vi "Test_ReadInconsistantSpreadsheet.vi"() -> ()   [LabVIEW 2014]
uses:
  functions/Timer_Global_Action_Control.ctl
panel:
  out "Time Difference 2":dbl
  out "Array Numeric":u8[](array[numeric])
  out "text":string
  out "Time Difference":dbl
  in  "type (empty)":string[][](array[string])
  out "all rows":string[][](array[string])
  # "10Mio Loops\n4,7sec"
  # "1k Loops:\nRaw: 0.0009999sec\nSmart: 14,1148sec"
  # "aa b   c\n\n#param1\tparam2\tparam3\tparam4\n!param5    param6\tparam7\tparam8\n\n1.00  1.20     1.30         1.40\n 2.00\t2.20\t2.30\t2.40\n3.00\t3.20\t3.30\t3.40\n     4.00    4.20   4.30 4.40"
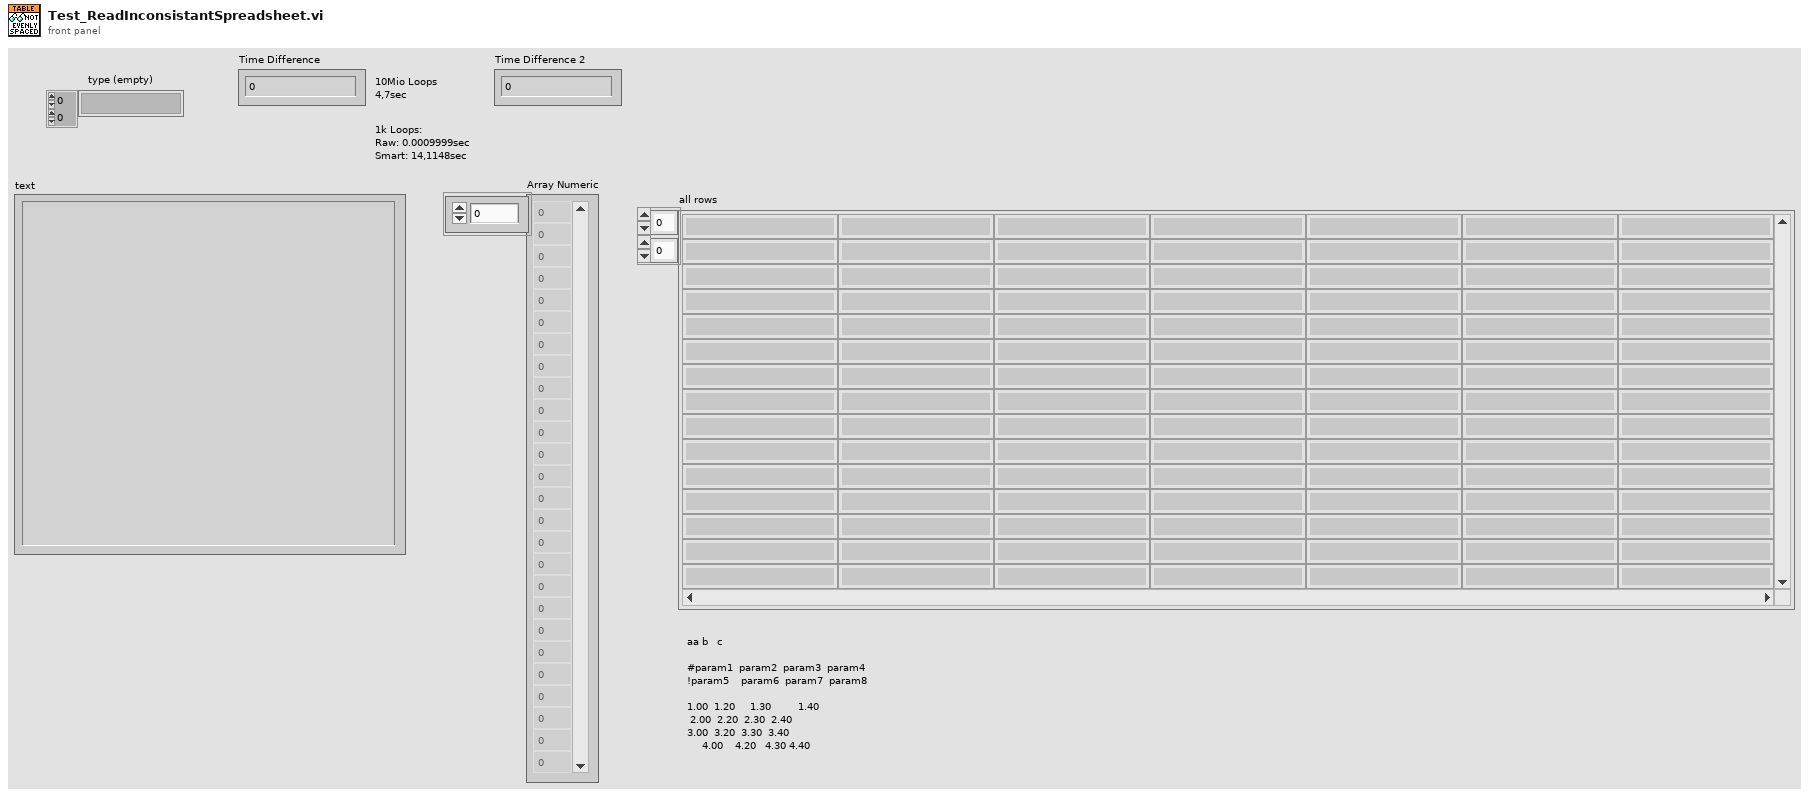
[diagram p1: front panel]
types:
  T1 = typedef "Timer_Global_Action_Control.ctl" = enum16{"Init", "Set", "Get", "Update", "Clear"}
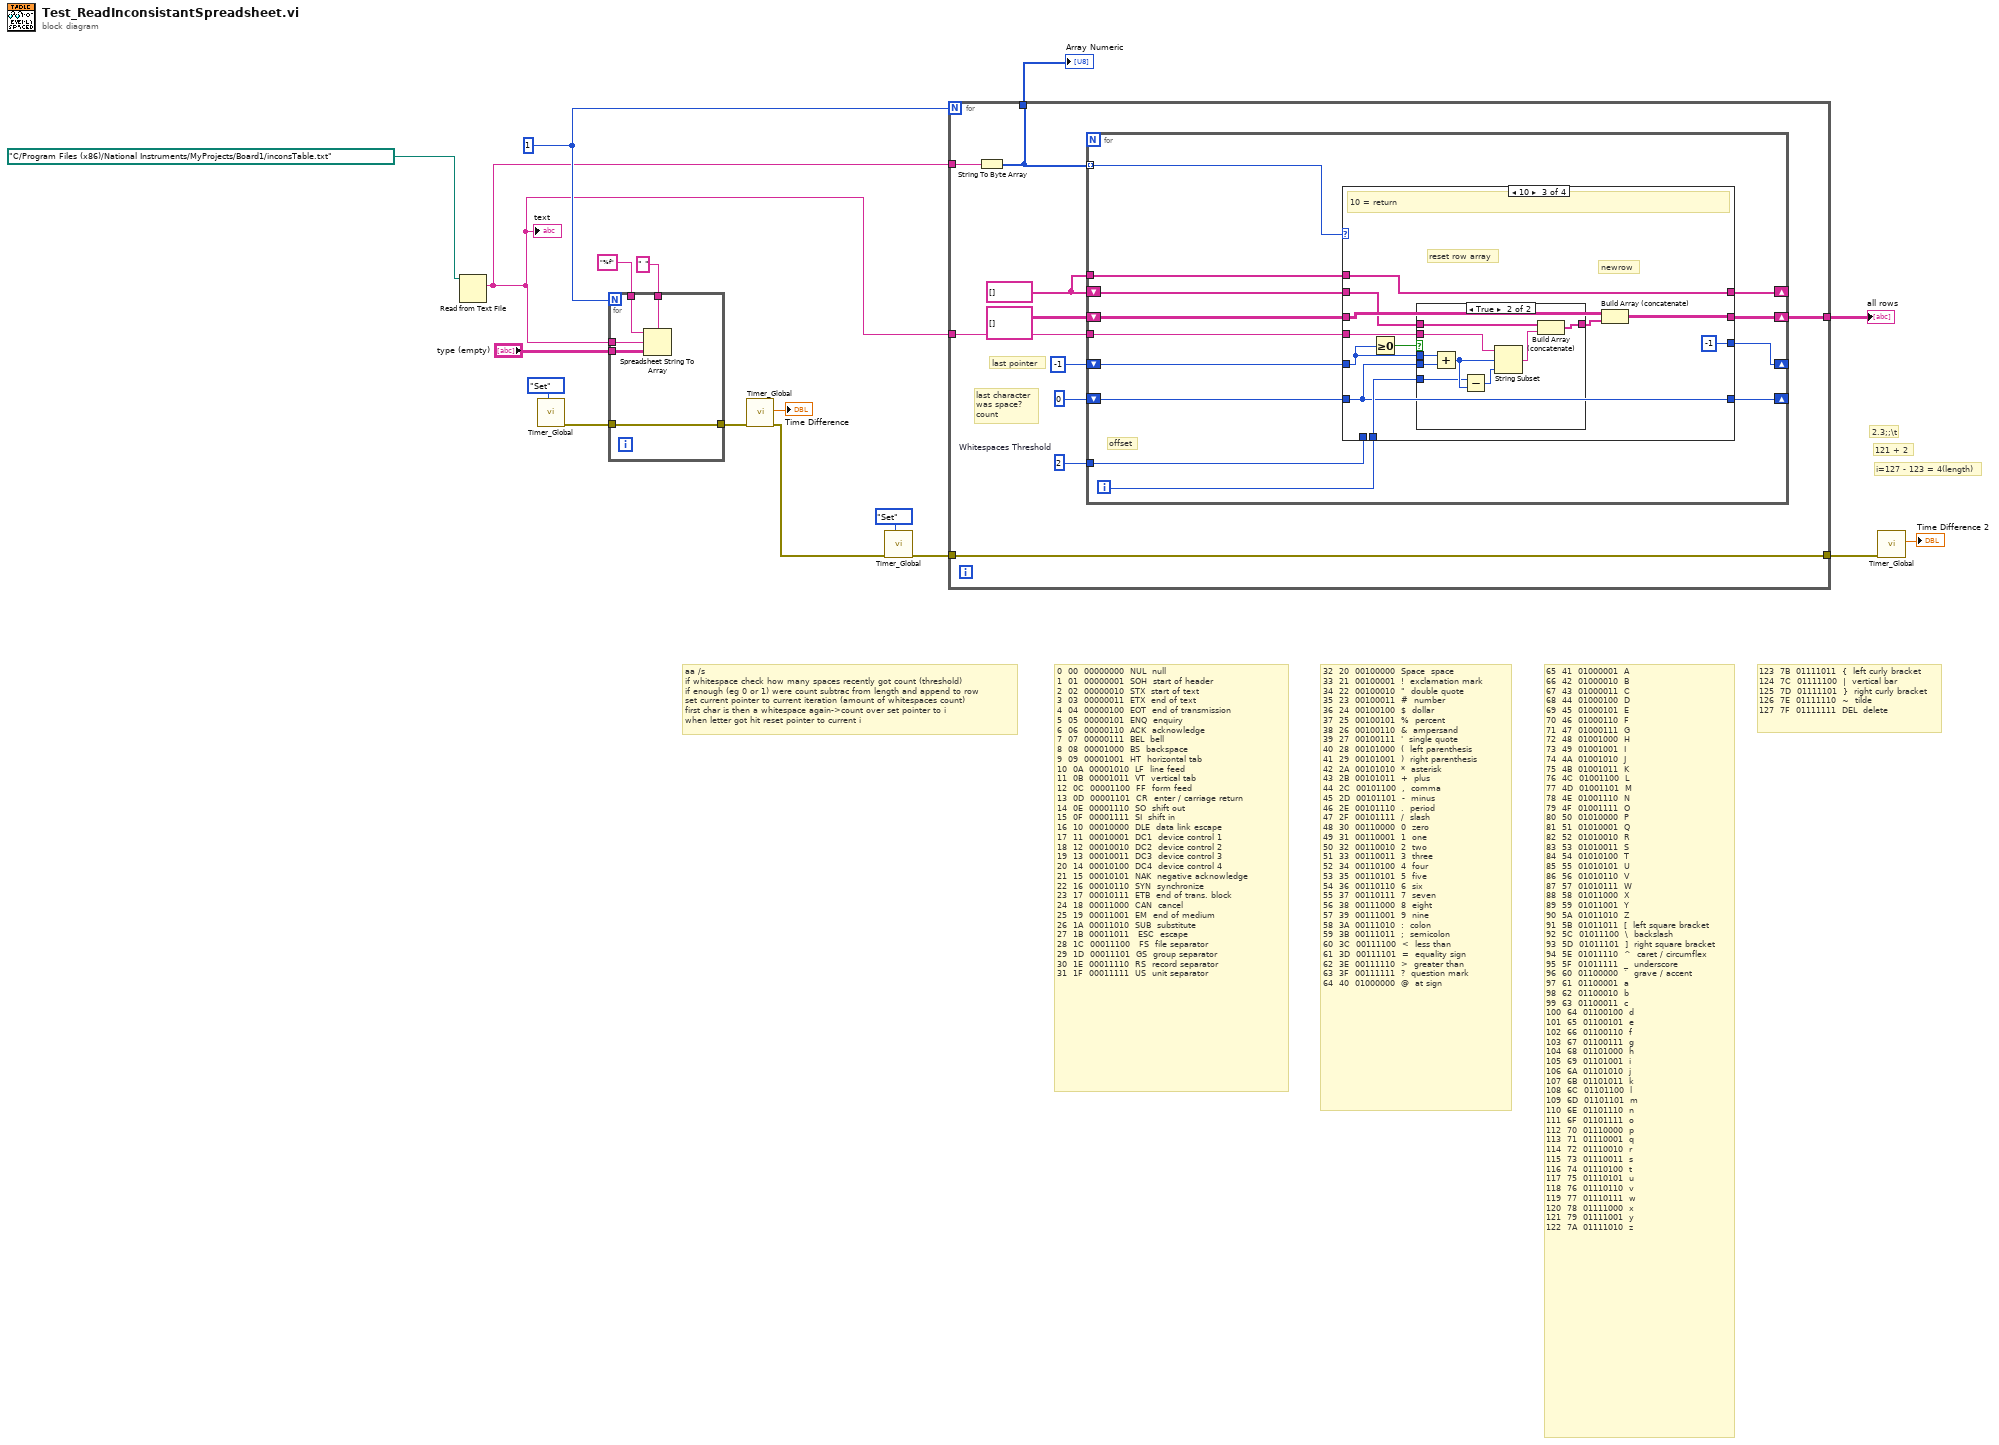
[diagram p0: block diagram]
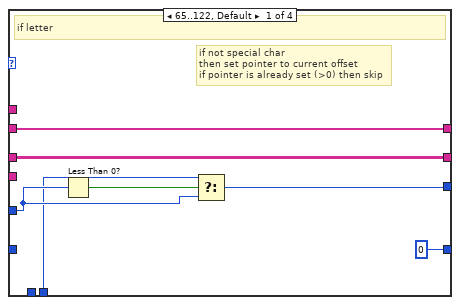
[diagram p2: hidden frame]
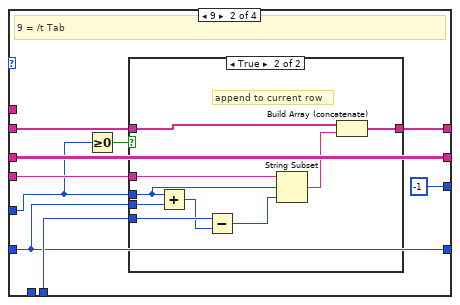
[diagram p3: hidden frame]
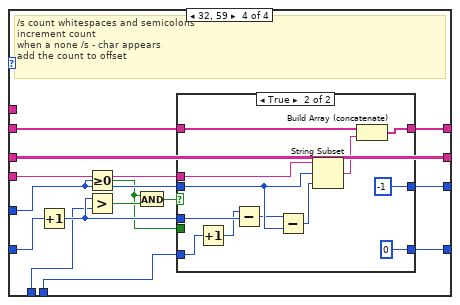
[diagram p6: hidden frame]
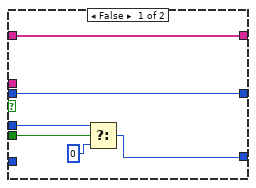
[diagram p7: hidden frame]
diagram:
  w3 = 1
  # "i=127 - 123 = 4(length)"
  # "121 + 2"
  # "2.3;;\\t"
  # "aa /s\nif whitespace check how many spaces recently got count (threshold)\nif enough (eg 0 or 1) were count subtrac from length and append to row\nset current pointer to current iteration (amount of whitespaces count)\nfirst char is then a whitespace again->count over set pointer to i\nwhen letter got hit reset pointer to current i"
  # "123 \t7B \t01111011 \t{ \tleft curly bracket\n124 \t7C \t01111100 \t| \tvertical bar\n125 \t7D \t01111101 \t} \tright curly bracket\n126 \t7E \t01111110 \t~ \ttilde\n127 \t7F \t01111111 \tDEL \tdelete"
  # "65 \t41 \t01000001 \tA \t \n66 \t42 \t01000010 \tB \t \n67 \t43 \t01000011 \tC \t \n68 \t44 \t01000100 \tD \t \n69 \t45 \t01000101 \tE \t \n70 \t46 \t01000110 \tF \t \n71 \t47 \t01000111 \tG \t \n72 \t48 \t01001000 \tH \t \n73 \t49 \t01001001 \tI \t \n74 \t4A \t01001010 \tJ \t \n75 \t4B \t01001011 \tK \t \n76 \t4C \t01001100 \tL \t \n77 \t4D \t01001101 \tM \t \n78 \t4E \t01001110 \tN \t \n79 \t4F \t01001111 \tO \t \n80 \t50 \t01010000 \tP \t \n81 \t51 \t01010001 \tQ \t \n82 \t52 \t01010010 \tR \t \n83 \t53 \t01010011 \tS \t \n84 \t54 \t01010100 \tT \t \n85 \t55 \t01010101 \tU \t \n86 \t56 \t01010110 \tV \t \n87 \t57 \t01010111 \tW \t \n88 \t58 \t01011000 \tX \t \n89 \t59 \t01011001 \tY \t \n90 \t5A \t01011010 \tZ \t \n91 \t5B \t01011011 \t[ \tleft square bracket\n92 \t5C \t01011100 \t\\ \tbackslash\n93 \t5D \t01011101 \t] \tright square bracket\n94 \t5E \t01011110 \t^ \tcaret / circumflex\n95 \t5F \t01011111 \t_ \tunderscore\n96 \t60 \t01100000 \t` \tgrave / accent\n97 \t61 \t01100001 \ta \t \n98 \t62 \t01100010 \tb \t \n99 \t63 \t01100011 \tc \t \n100 \t64 \t01100100 \td \t \n101 \t65 \t01100101 \te \t \n102 \t66 \t01100110 \tf \t \n103 \t67 \t01100111 \tg \t \n104 \t68 \t01101000 \th \t \n105 \t69 \t01101001 \ti \t \n106 \t6A \t01101010 \tj \t \n107 \t6B \t01101011 \tk \t \n108 \t6C \t01101100 \tl \t \n109 \t6D \t01101101 \tm \t \n110 \t6E \t01101110 \tn \t \n111 \t6F \t01101111 \to \t \n112 \t70 \t01110000 \tp \t \n113 \t71 \t01110001 \tq \t \n114 \t72 \t01110010 \tr \t \n115 \t73 \t01110011 \ts \t \n116 \t74 \t01110100 \tt \t \n117 \t75 \t01110101 \tu \t \n118 \t76 \t01110110 \tv \t \n119 \t77 \t01110111 \tw \t \n120 \t78 \t01111000 \tx \t \n121 \t79 \t01111001 \ty \t \n122 \t7A \t01111010 \tz"
  # "32 \t20 \t00100000 \tSpace \tspace\n33 \t21 \t00100001 \t! \texclamation mark\n34 \t22 \t00100010 \t\" \tdouble quote\n35 \t23 \t00100011 \t# \tnumber\n36 \t24 \t00100100 \t$ \tdollar\n37 \t25 \t00100101 \t% \tpercent\n38 \t26 \t00100110 \t& \tampersand\n39 \t27 \t00100111 \t' \tsingle quote\n40 \t28 \t00101000 \t( \tleft parenthesis\n41 \t29 \t00101001 \t) \tright parenthesis\n42 \t2A \t00101010 \t* \tasterisk\n43 \t2B \t00101011 \t+ \tplus\n44 \t2C \t00101100 \t, \tcomma\n45 \t2D \t00101101 \t- \tminus\n46 \t2E \t00101110 \t. \tperiod\n47 \t2F \t00101111 \t/ \tslash\n48 \t30 \t00110000 \t0 \tzero\n49 \t31 \t00110001 \t1 \tone\n50 \t32 \t00110010 \t2 \ttwo\n51 \t33 \t00110011 \t3 \tthree\n52 \t34 \t00110100 \t4 \tfour\n53 \t35 \t00110101 \t5 \tfive\n54 \t36 \t00110110 \t6 \tsix\n55 \t37 \t00110111 \t7 \tseven\n56 \t38 \t00111000 \t8 \teight\n57 \t39 \t00111001 \t9 \tnine\n58 \t3A \t00111010 \t: \tcolon\n59 \t3B \t00111011 \t; \tsemicolon\n60 \t3C \t00111100 \t< \tless than\n61 \t3D \t00111101 \t= \tequality sign\n62 \t3E \t00111110 \t> \tgreater than\n63 \t3F \t00111111 \t? \tquestion mark\n64 \t40 \t01000000 \t@ \tat sign"
  # "0 \t00 \t00000000 \tNUL \tnull\n1 \t01 \t00000001 \tSOH \tstart of header\n2 \t02 \t00000010 \tSTX \tstart of text\n3 \t03 \t00000011 \tETX \tend of text\n4 \t04 \t00000100 \tEOT \tend of transmission\n5 \t05 \t00000101 \tENQ \tenquiry\n6 \t06 \t00000110 \tACK \tacknowledge\n7 \t07 \t00000111 \tBEL \tbell\n8 \t08 \t00001000 \tBS \tbackspace\n9 \t09 \t00001001 \tHT \thorizontal tab\n10 \t0A \t00001010 \tLF \tline feed\n11 \t0B \t00001011 \tVT \tvertical tab\n12 \t0C \t00001100 \tFF \tform feed\n13 \t0D \t00001101 \tCR \tenter / carriage return\n14 \t0E \t00001110 \tSO \tshift out\n15 \t0F \t00001111 \tSI \tshift in\n16 \t10 \t00010000 \tDLE \tdata link escape\n17 \t11 \t00010001 \tDC1 \tdevice control 1\n18 \t12 \t00010010 \tDC2 \tdevice control 2\n19 \t13 \t00010011 \tDC3 \tdevice control 3\n20 \t14 \t00010100 \tDC4 \tdevice control 4\n21 \t15 \t00010101 \tNAK \tnegative acknowledge\n22 \t16 \t00010110 \tSYN \tsynchronize\n23 \t17 \t00010111 \tETB \tend of trans. block\n24 \t18 \t00011000 \tCAN \tcancel\n25 \t19 \t00011001 \tEM \tend of medium\n26 \t1A \t00011010 \tSUB \tsubstitute\n27 \t1B \t00011011 \t ESC \tescape\n28 \t1C \t00011100 \t FS \tfile separator\n29 \t1D \t00011101 \tGS \tgroup separator\n30 \t1E \t00011110 \tRS \trecord separator\n31 \t1F \t00011111 \tUS \tunit separator"
  n1 = Read from Text File(file (use dialog)=path "C:/Program Files (x86)/National Instruments/MyProjects/Board1/inconsTable.txt" ("Open File")) -> (text=w2:string)  [unwired: 3 in, 3 out]
  "text" <- w2
  n2 = call "Timer_Global.vi"("Timer Action"=Timer_Global_Action_Control."Set") -> ("Error Out"=w15:errorcluster)  [unwired: 8 in, 2 out]
  n3 = for {
    N: w3 -> [_]
    tunnel: "type (empty)" -> [w22]
    tunnel: w2 -> [w19]
    tunnel: [w21] -> w14
    tunnel: w15 -> [w21]
    tunnel: " " ("delimiter (\\t)") -> [w20]
    tunnel: "%f" ("format (%s)") -> [w18]
    n4 = Spreadsheet String To Array(delimiter (Tab)=w20, format string=w18, spreadsheet string=w19, array type (2D Dbl)=w22) -> ()  [unwired: 1 out]
  }
  n5 = call "Timer_Global.vi"("Error In"=w14) -> ("Error Out"=w7:errorcluster, "Time Difference"=→"Time Difference":dbl)  [unwired: 8 in, 1 out]
  n6 = call "Timer_Global.vi"("Timer Action"=Timer_Global_Action_Control."Set", "Error In"=w7) -> ("Error Out"=w4:errorcluster)  [unwired: 7 in, 2 out]
  n7 = for {
    N: w3 -> [_]
    tunnel: [w32] -> w9
    tunnel: w2 -> [w27]
    tunnel: [w25] -> w5
    tunnel: w4 -> [w25]
    tunnel: w2 -> [w24]
    tunnel: [w23] -> w1
    w26 = 2  # Whitespaces Threshold
    w30 = string[] [] ("all rows 2")
    # "last pointer"
    # "last character\nwas space?\ncount"
    n8 = String To Byte Array(string=w24) -> (unsigned byte array=w23:u8[])
    n9 = for {
      tunnel: w23 -> [w40] mode=indexing
      shift-right: [w44] -> w32
      shift-left: string[][] [] ("all rows 2") -> [w45]
      shift-right: [w41] -> _
      shift-left: w30 -> [w43]
      tunnel: w30 -> [w42]
      shift-right: [w35] -> _
      shift-left: 0 ("y") -> [w34]
      shift-right: [w37] -> _
      shift-left: -1 ("y") -> [w39]
      tunnel: w27 -> [w36]
      tunnel: w26 -> [w33]
      i -> [w38]
      # "offset"
      n10 = case shown="10" w40 {
        tunnel: w45 -> [w52 w59 w82 w106]
        tunnel: [w52 w59 w81 w106] -> w44
        tunnel: w43 -> [w51 w61 w79 w102]
        tunnel: w42 -> [_ _ w80 _]
        tunnel: [w51 w60 w80 w101] -> w41
        tunnel: w39 -> [w50 w55 w73 w94]
        tunnel: w38 -> [w48 w56 w76 w99]
        tunnel: [w49 -1 ("y") -1 ("y") w100] -> w37
        tunnel: w36 -> [_ w58 w75 w103]
        tunnel: [0 ("y") w53 w72 w104] -> w35
        tunnel: w34 -> [_ w53 w72 w105]
        tunnel: w33 -> [_ _ _ w97]
        frame 65..122, Default {
          # "if not special char\nthen set pointer to current offset\nif pointer is already set (>0) then skip"
          # "if letter"
          n11 = Less Than 0?(x=w50) -> (x < 0?=w47:bool)
          n12 = Select(t=w48, s=w47, f=w50) -> (s? t:f=w49:i32)
        }
        frame 9 {
          # "9 = /t Tab"
          n13 = Greater Or Equal To 0?(x=w55) -> (x >= 0?=w54:bool)
          n14 = case shown="True" w54 {
            tunnel: w61 -> [w62 w71]
            tunnel: [w62 w70] -> w60
            tunnel: w58 -> [_ w69]
            tunnel: w56 -> [_ w66]
            tunnel: w53 -> [_ w64]
            tunnel: w55 -> [_ w63]
            frame False {
            }
            frame True {
              # "append to current row"
              n15 = Add(x=w63, y=w64) -> (x+y=w65:i32)
              n16 = Subtract(x=w66, y=w65) -> (x-y=w67:i32)
              n17 = String Subset(string=w69, offset (0)=w63, length (rest)=w67) -> (substring=w68:string)
              n18 = Build Array (concatenate)(w71, w68) -> (w70:string[])
            }
          }
        }
        frame 10 {
          # "reset row array"
          # "newrow"
          # "10 = return"
          n19 = Greater Or Equal To 0?(x=w73) -> (x >= 0?=w74:bool)
          n20 = case shown="True" w74 {
            tunnel: w79 -> [w83 w90]
            tunnel: [w83 w89] -> w78
            tunnel: w72 -> [_ w87]
            tunnel: w73 -> [_ w86]
            tunnel: w76 -> [_ w85]
            tunnel: w75 -> [_ w84]
            frame False {
            }
            frame True {
              n21 = Add(x=w86, y=w87) -> (x+y=w91:i32)
              n22 = Subtract(x=w85, y=w91) -> (x-y=w92:i32)
              n23 = String Subset(string=w84, offset (0)=w91, length (rest)=w92) -> (substring=w88:string)
              n24 = Build Array (concatenate)(w90, w88) -> (w89:string[])
            }
          }
          n25 = Build Array (concatenate)(w82, w78) -> (w81:string[][])
        }
        frame 32, 59 {
          # "/s count whitespaces and semicolons\nincrement count\nwhen a none /s - char appears\nadd the count to offset"
          n26 = Increment(x=w105) -> (x+1=w98:i32)
          n27 = Greater Or Equal To 0?(x=w94) -> (x >= 0?=w93:bool)
          n28 = Greater?(x=w98, y=w97) -> (0:w95:bool)
          n29 = And(x=w93, y=w95) -> (x .and. y?=w96:bool)
          n30 = case shown="True" w96 {
            tunnel: [w108 0 ("y")] -> w104
            tunnel: w98 -> [w107 w117]
            tunnel: w103 -> [_ w123]
            tunnel: w102 -> [w112 w122]
            tunnel: [w112 w121] -> w101
            tunnel: [w111 -1 ("y")] -> w100
            tunnel: w94 -> [w111 w118]
            tunnel: w99 -> [_ w114]
            tunnel: w93 -> [w109 _]
            frame False {
              n31 = Select(t=w107, s=w109, f=0 ("y")) -> (s? t:f=w108:i32)
            }
            frame True {
              n32 = Increment(x=w114) -> (x+1=w113:i32)
              n33 = Subtract(x=w113, y=w117) -> (x-y=w116:i32)
              n34 = Subtract(x=w116, y=w118) -> (x-y=w119:i32)
              n35 = String Subset(string=w123, offset (0)=w118, length (rest)=w119) -> (substring=w120:string)
              n36 = Build Array (concatenate)(w122, w120) -> (w121:string[])
            }
          }
        }
      }
    }
  }
  "Array Numeric" <- w1
  "all rows" <- w9
  n37 = call "Timer_Global.vi"("Error In"=w5) -> ("Time Difference"=→"Time Difference 2":dbl)  [unwired: 8 in, 2 out]
